vi "LeonardoJoystick.vi"() -> ()   [LabVIEW 2014]
panel:
  out "buttons":bool[](array[boolean])
  in  "stop":bool
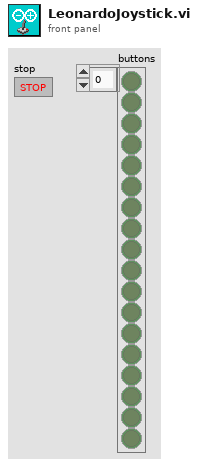
[diagram p1: front panel]
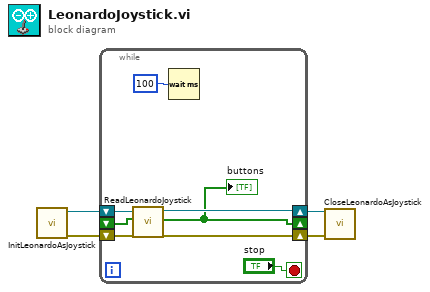
[diagram p0: block diagram]
diagram:
  n1 = call "InitLeonardoAsJoystick.vi"() -> ("error out"=w3:errorcluster, "Refnum out"=w4:refnum<k1>)  [unwired: 10 in]
  n2 = while {
    shift-right: [w10] -> w2
    shift-left: w4 -> [w12]
    shift-right: [w9] -> w1
    shift-left: w3 -> [w11]
    shift-right: [w6] -> _
    shift-left: _ -> [w5]
    stop <- "stop" stop-if-true
    n3 = call "ReadLeonardoJoystick.vi"("error in (no error)"=w11, "Previous buttons"=w5, "Refnum in"=w12) -> ("error out"=w9:errorcluster, "buttons"=w6:bool[], "Refnum out"=w10:refnum<k1>)  [unwired: 6 in]
    "buttons" <- w6
    n4 = Wait (ms)(milliseconds to wait=u32 100) -> ()  [unwired: 1 out]
  }
  n5 = call "CloseLeonardoAsJoystick.vi"("error in (no error)"=w1, "Refnum in"=w2) -> ()  [unwired: 10 in]
